vi "Excit_Extract_Fs.vi"(8 "error in (no error)":errorcluster, 11 "EXCIT Inputs":T1={"Number of Excitations"=1, "Script Text"="", "Table of Waveforms"=[]} {"Number of Excitations" min=1 max=10}) -> (0 "error out":errorcluster caption="sortie d'erreur", 2 "Sample Rate":dbl)   [LabVIEW 2017]
doc: "From a start and end value, generates an adiabatic waveform signal of 2000 values (double).\nWrites this waveform into a binary file, in a big-endian format.\nDisplays the written data and the FFT of the signal.\nDefault Path for the generated file is D:\\PIRENEA\\EXCIT_WFMS\n\nAvailable Waveforms : Sinus, Swift, Chirp, Ramp (Up or Down), DoubleRamp (Up-Down or Down-Up)"
uses:
  controls/EXCIT_Inputs.ctl
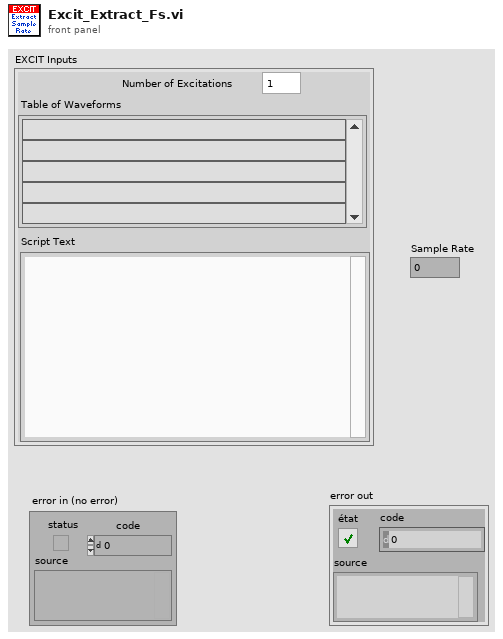
[diagram p1: front panel]
types:
  T1 = typedef "EXCIT_Inputs.ctl" = cluster{"Number of Excitations":i32, "Script Text":string, "Table of Waveforms":string[]}
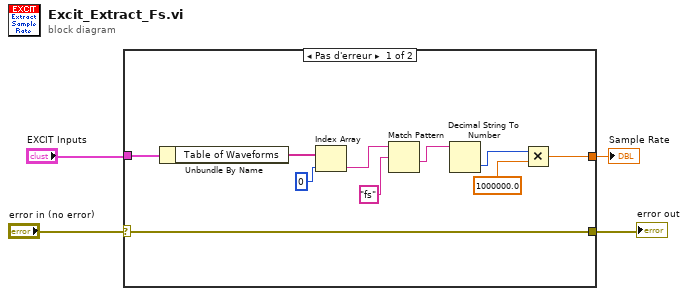
[diagram p0: block diagram]
diagram:
  n1 = case shown="Pas d'erreur" "error in (no error)" {
    selector: "error in (no error)" -> [w6 w15]
    tunnel: [w6 w15] -> w4
    tunnel: "EXCIT Inputs" -> [w7 _]
    tunnel: [w5 _] -> w2
    frame No Error {
      n2 = Unbundle By Name(w7) -> ("Table of Waveforms"=w14:string[])
      n3 = Index Array(array=w14, index=0 ("indice")) -> (element=w12:string)
      n4 = Match Pattern(string=w12, regular expression="fs" ("expression régulière")) -> (after substring=w10:string)  [unwired: 1 in, 3 out]
      n5 = Decimal String To Number(string=w10) -> (number=w9:i32)  [unwired: 2 in, 1 out]
      n6 = Multiply(x=w9, y=1000000.0) -> (x*y=w5:dbl)
    }
    frame Error {
    }
  }
  "error out" <- w4
  "Sample Rate" <- w2
